vi "Flow Set P&F.vi"() -> ()   [LabVIEW 2017]
panel:
  out "Flow Set":dbl
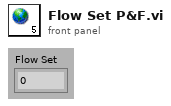
[diagram p1: front panel]
diagram:
